vi "Start Feeder Implementation.vi"(8 "Deadband (RPM)":dbl, 10 "Velocity Setpoint In":dbl, 11 "Feeder":T1) -> (0 "Finished?":bool, 3 "Velocity Setpoint Out":dbl)   [LabVIEW 2019]
uses:
  <vilib>/Rock Robotics/WPI/MotorControl/WPI_MotorControlDeviceRef.ctl
  <vilib>/Rock Robotics/WPI/MotorControl/WPI_MotorControlType.ctl
  <vilib>/Rock Robotics/SystemInterfaces/DIO/FPGA_DIOPWMChannel.ctl
  <vilib>/Rock Robotics/WPI/PWM/WPI_PWMDeadband.ctl
  <vilib>/Rock Robotics/SystemInterfaces/DIO/FPGA_DIOChannel.ctl
  Feeder Published Globals.vi
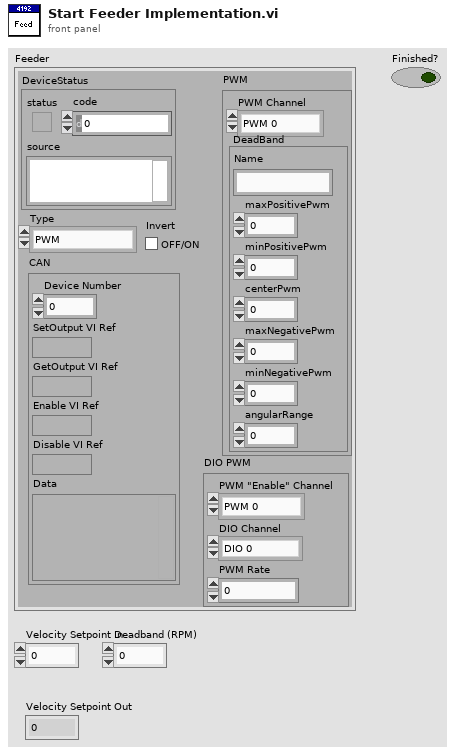
[diagram p1: front panel]
types:
  T1 = typedef "WPI_MotorControlDeviceRef.ctl" = cluster{"DeviceStatus":errorcluster, "Type":T2, "PWM":cluster{"PWM Channel":T3, "DeadBand":T4}, "CAN":cluster{"Device Number":u8, "SetOutput VI Ref":variant, "GetOutput VI Ref":variant, "Enable VI Ref":variant, "Disable VI Ref":variant, "Data":variant}, "Invert":bool, "DIO PWM":cluster{"PWM \"Enable\" Channel":T3, "DIOChannel":T5, "PWM Rate":dbl}}
  T2 = typedef "WPI_MotorControlType.ctl" = enum16{"PWM", "CAN", "DIO PWM"}
  T3 = typedef "FPGA_DIOPWMChannel.ctl" = enum8{"PWM 0", "PWM 1", "PWM 2", "PWM 3", "PWM 4", "PWM 5", "PWM 6", "PWM 7", "PWM 8", "PWM 9", "PWM MXP 0", "PWM MXP 1", "PWM MXP 2", "PWM MXP 3", "PWM MXP 4", "PWM MXP 5", "PWM MXP 6", "PWM MXP 7", "PWM MXP 8", "PWM MXP 9", "Invalid"}
  T4 = typedef "WPI_PWMDeadband.ctl" = cluster{"Name":string, "maxPositivePwm":i32, "minPositivePwm":i32, "centerPwm":i32, "maxNegativePwm":i32, "minNegativePwm":i32, "angularRange":u16}
  T5 = typedef "FPGA_DIOChannel.ctl" = enum8{"DIO 0", "DIO 1", "DIO 2", "DIO 3", "DIO 4", "DIO 5", "DIO 6", "DIO 7", "DIO 8", "DIO 9", "DIO MXP 0", "DIO MXP 1", "DIO MXP 2", "DIO MXP 3", "DIO MXP 4", "DIO MXP 5", "DIO MXP 6", "DIO MXP 7", "DIO MXP 8", "DIO MXP 9", "DIO MXP 10", "DIO MXP 11", "DIO MXP 12", "DIO MXP 13", "DIO MXP 14", "DIO MXP 15", "SPI Port CS1", "SPI Port CS2", "SPI Port CS3", "SPI Port MISO", "SPI Port MOSI", "Invalid"}
  T6 = cluster{"Feeder Velocity":cluster{"Sensor Velocity":dbl, "Setpoint":dbl, "Applied Output":dbl}, "Feeder PID Constants":cluster{"P Gain":dbl, "I Gain":dbl, "D Gain":dbl, "F Gain":dbl, "I Zone":dbl, "Min Output":dbl, "Max Output":dbl}}
  T7 = cluster{"P Gain":dbl, "I Gain":dbl, "D Gain":dbl, "F Gain":dbl, "I Zone":dbl, "Min Output":dbl, "Max Output":dbl}
  T8 = cluster{dbl, "Velocity Setpoint In":dbl, "Applied Output":dbl}
  T9 = cluster{"Feeder Up To Speed? ":bool, "Index Clear?":bool}
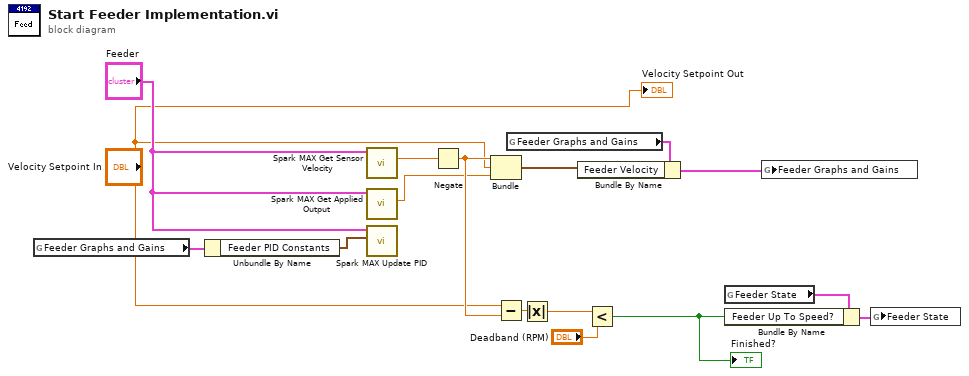
[diagram p0: block diagram]
diagram:
  n1 = global read "Feeder Published Globals.vi" "Feeder Graphs and Gains"() -> (w2:T6)
  n2 = Unbundle By Name(w2) -> ("Feeder PID Constants"=w1:T7)
  n3 = call <vilib>:"Spark MAX Get Sensor Velocity.vi"("MotorControlDevRef in"="Feeder") -> ("Sensor Velocity"=w13:dbl)  [unwired: 7 in, 3 out]
  n4 = call <vilib>:"Spark MAX Get Applied Output.vi"("MotorControlDevRef in"="Feeder") -> ("Applied Output"=w11:dbl)  [unwired: 7 in, 3 out]
  n5 = call "Spark MAX Update PID.vi"("MotorControlDeviceRef"="Feeder", "PID Constants"=w1) -> ()  [unwired: 8 in]
  n6 = Negate(x=w13) -> (-x=w14:dbl)
  n7 = Bundle(w14, "Velocity Setpoint In"="Velocity Setpoint In", "Applied Output"=w11) -> (w3:T8)  [unwired: 1 in]
  n8 = Subtract(x="Velocity Setpoint In", y=w14) -> (x-y=w15:dbl)
  n9 = global read "Feeder Published Globals.vi" "Feeder Graphs and Gains"() -> (w5:T6)
  n10 = Absolute Value(x=w15) -> (abs(x)=w16:dbl)
  n11 = Bundle By Name(cluster=w5, "Feeder Velocity"=w3) -> (w4:T6)
  n12 = Less?(x=w16, y="Deadband (RPM)") -> (x < y?=w6:bool)
  "Finished?" <- w6
  n13 = global read "Feeder Published Globals.vi" "Feeder State"() -> (w7:T9)
  n14 = Bundle By Name(cluster=w7, "Feeder Up To Speed?"=w6) -> (w8:T9)
  n15 = global write "Feeder Published Globals.vi" "Feeder Graphs and Gains"(w4) -> ()
  n16 = global write "Feeder Published Globals.vi" "Feeder State"(w8) -> ()
  "Velocity Setpoint Out" <- "Velocity Setpoint In"
